vi "GlobalCamHandle.vi"() -> ()   [LabVIEW 2010]
panel:
  in  "Camera Handle":u32
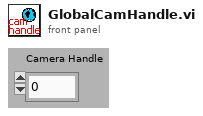
[diagram p1: front panel]
diagram:
